vi "Create.vi"(8 "ErrorIn":errorcluster, 11 "ReferenceIn":refnum<class "TemplateGUI.lvclass">) -> (0 "ErrorOut":errorcluster, 3 "ReferenceOut":refnum<class "TemplateGUI.lvclass">)   [LabVIEW 2021, in "TemplateGUIOpenGDSActiveObject.lvlib" / "TemplateGUI.lvclass"]
doc: "Create the object instance"
uses:
  TemplateGUI.lvclass
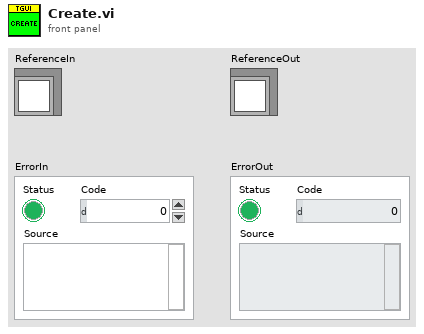
[diagram p1: front panel]
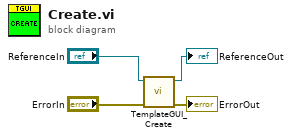
[diagram p0: block diagram]
diagram:
  n1 = call "TemplateGUI_Create.vi"("ErrorIn"="ErrorIn", "ReferenceIn"="ReferenceIn") -> ("ErrorOut"=→"ErrorOut":errorcluster, "ReferenceOut"=→"ReferenceOut":refnum<class "TemplateGUI.lvclass">)  [unwired: 8 in]
